vi "cRIO_triggered_laser_log.vi"() -> ()   [LabVIEW 2020]
uses:
  <vilib>/Platform/TimedLoop/XDataNode/timing_clust.ctl
  <vilib>/Platform/TimedLoop/XDataNode/nitl_modes.ctl
  <vilib>/Platform/TimedLoop/XDataNode/wakeup.ctl
  <vilib>/Utility/file.llb/Write Delimited Spreadsheet (DBL).vi
  <vilib>/Platform/TimedLoop/XDataNode/loadnilvce.vi
  <vilib>/platform/TimedLoop/XDataNode/XDataNode.xnode
  <vilib>/Platform/TimedLoop/XDataNode/XDNodeRunTimeDep.lvlib
panel:
  out "Laser Displacement - cRIO (onboard execution)":dbl[][](graph)
  out "Readout (V)":dbl[][](array[numeric])
  out "Laser Displacement - cRIO (logged data)":dbl[][](graph)
  in  "stop":bool
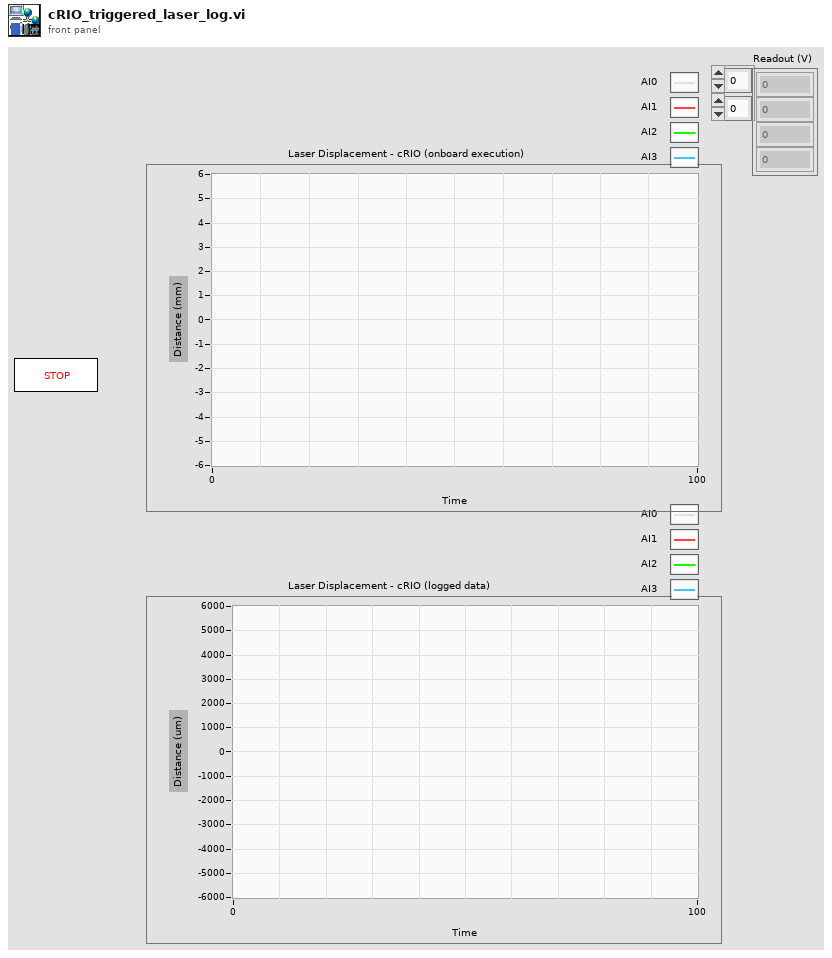
[diagram p1: front panel]
types:
  T1 = typedef "XDNodeRunTimeDep.lvlib/timing_clust.ctl" = cluster{"Expected End [f-1]":u64, "Actual End [f-1]":u64, "Finished Late? [f-1]":bool, "Expected End [i-1]":u64, "Actual End [i-1]":u64, "Finished Late? [i-1]":bool, "Expected Start [i]":u64, "Actual Start [i]":u64, "Expected Start [f]":u64, "Actual Start [f]":u64, "Source Name":string, "Structure Name":string, "Period":i64, "Deadline":i64, "Offset":i64, "Start":i64, "Priority":i32, "Timeout":i32, "Mode":T2, "Wakeup Reason":T3, "Error":errorcluster, "Source Type":string, "Secondary Source Type":string, "Global End Time":u64, "Global Start Time":u64, "Frame Duration":u64, "Iteration Duration":u64, "Assigned CPU":i32, "I/O Scan Engine Mode":u32}
  T2 = typedef "XDNodeRunTimeDep.lvlib/nitl_modes.ctl" = enum32{"No Change", "Process missed periods, maintain original phase", "Discard missed periods, maintain original phase", "Process missed periods, ignore original phase", "Discard missed periods, ignore original phase"}
  T3 = typedef "XDNodeRunTimeDep.lvlib/wakeup.ctl" = enum32{"Normal", "Aborted", "Asynchronous wakeup", "Timing source error", "Timed loop error", "Timeout"}
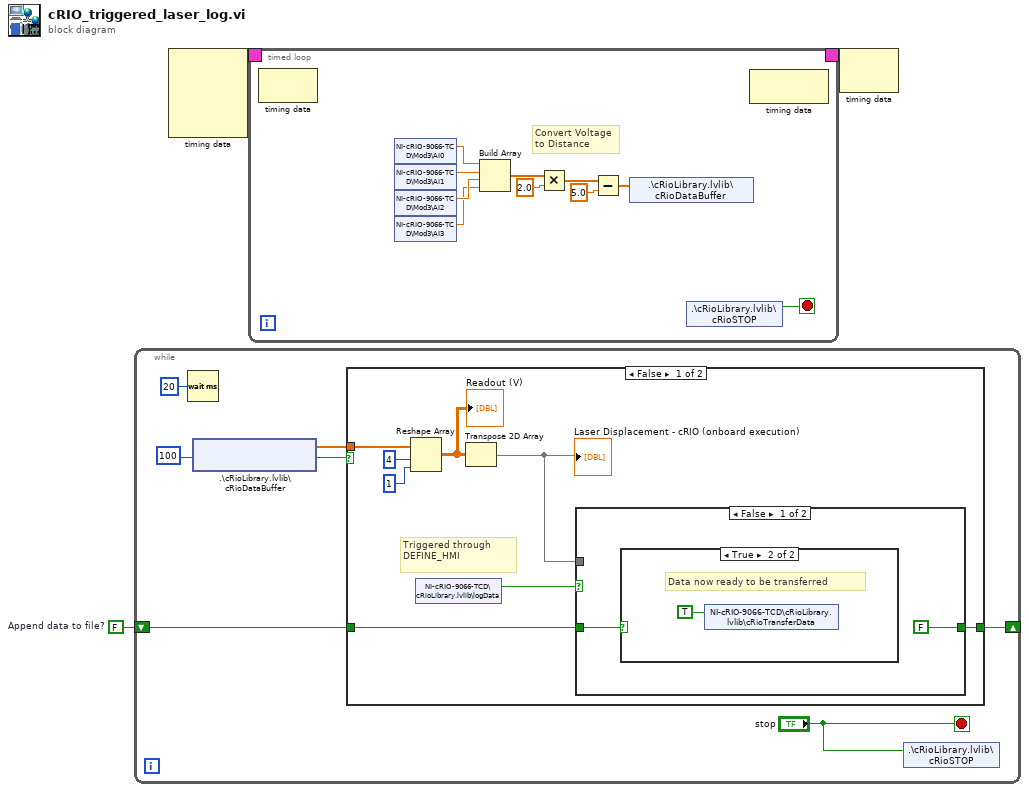
[diagram p0: block diagram]
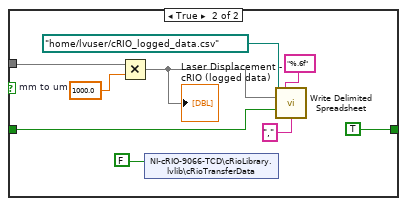
[diagram p3: hidden frame]
diagram:
  w1 = FALSE  # Append data to file?
  n1 = while {
    shift-right: [w10] -> _
    shift-left: w1 -> [w9]
    stop <- "stop" stop-if-true
    n2 = Wait (ms)(milliseconds to wait=u32 20) -> ()  [unwired: 1 out]
    n3 = shared-variable ".\\cRioLibrary.lvlib\\cRioDataBuffer"(100) -> (w7:dbl[], w6:bool)  [unwired: 1 in, 1 out]
    n4 = case shown="False" w6 {
      tunnel: w7 -> [w13 _]
      tunnel: [w14 w31] -> w10
      tunnel: w9 -> [w18 w31]
      frame False {
        # "Triggered through \nDEFINE_HMI"
        n5 = Reshape Array(w13, 4 ("dimension size"), 1 ("dimension size")) -> (w15:dbl[][])
        "Readout (V)" <- w15
        n6 = shared-variable "NI-cRIO-9066-TCD\\cRioLibrary.lvlib\\logData"() -> (w11:bool)  [unwired: 1 in, 1 out]
        n7 = Transpose 2D Array(2D array=w15) -> (transposed array=w12:dbl[][])
        "Laser Displacement - cRIO (onboard execution)" <- w12
        n8 = case shown="False" w11 {
          tunnel: w18 -> [w19 w25]
          tunnel: w12 -> [_ w29]
          tunnel: [FALSE TRUE] -> w14
          frame False {
            n9 = case shown="True" w19 {
              frame False {
                # "Do nothing with Data"
              }
              frame True {
                # "Data now ready to be transferred"
                n10 = shared-variable "NI-cRIO-9066-TCD\\cRioLibrary.lvlib\\cRioTransferData"(TRUE) -> ()  [unwired: 1 in, 1 out]
              }
            }
          }
          frame True {
            w30 = 1000.0  # mm to um
            n11 = Multiply(x=w29, y=w30) -> (x*y=w23:dbl[][])
            "Laser Displacement - cRIO (logged data)" <- w23
            n12 = shared-variable "NI-cRIO-9066-TCD\\cRioLibrary.lvlib\\cRioTransferData"(FALSE) -> ()  [unwired: 1 in, 1 out]
            n13 = call-poly <vilib>:"Write Delimited Spreadsheet.vi"("file path (dialog if empty)"=path "/home/lvuser/cRIO_logged_data.csv", "format (%.3f)"="%.6f", "2D data"=w23, "append to file? (new file:F)"=w25, "delimiter (\\t)"="," ("delimiter (\\t)")) -> ()  [unwired: 9 in, 2 out]
          }
        }
      }
      frame True {
        # "Timed out - no data in buffer to process"
      }
    }
    n14 = shared-variable ".\\cRioLibrary.lvlib\\cRioSTOP"("stop") -> ()  [unwired: 1 in, 1 out]
  }
  n15 = node-c288() -> (w3:T1)  [unwired: 4 in]
  n16 = timed-loop {
    timing: w3 -> [_]
    timing-out: [_] -> w2
    stop <- w41 stop-if-true
    # "Convert Voltage to Distance"
    n17 = node-c288() -> ()  [unwired: 1 in, 1 out]
    n18 = shared-variable "NI-cRIO-9066-TCD\\Mod3\\AI0"() -> (w37:dbl)  [unwired: 1 in, 1 out]
    n19 = shared-variable "NI-cRIO-9066-TCD\\Mod3\\AI1"() -> (w34:dbl)  [unwired: 1 in, 1 out]
    n20 = shared-variable "NI-cRIO-9066-TCD\\Mod3\\AI2"() -> (w36:dbl)  [unwired: 1 in, 1 out]
    n21 = shared-variable "NI-cRIO-9066-TCD\\Mod3\\AI3"() -> (w35:dbl)  [unwired: 1 in, 1 out]
    n22 = Build Array(w37, w34, w36, w35) -> (w32:dbl[])
    n23 = Multiply(x=w32, y=2.0) -> (x*y=w39:dbl[])
    n24 = Subtract(x=w39, y=5.0) -> (x-y=w33:dbl[])
    n25 = shared-variable ".\\cRioLibrary.lvlib\\cRioDataBuffer"(w33) -> ()  [unwired: 1 in, 1 out]
    n26 = shared-variable ".\\cRioLibrary.lvlib\\cRioSTOP"() -> (w41:bool)  [unwired: 1 in, 1 out]
    n27 = node-c288() -> ()  [unwired: 1 in, 1 out]
  }
  n28 = node-c288(w2) -> ()  [unwired: 1 out]
